vi "RSZVB Trace Response Data Error.vi"(8 "error in (no error)":errorcluster {"code" format="%.0x"}, 9 "Error Term (1)":i32=1, 10 "Channel (Trace) (1)":i32=1, 11 "VISA session":refnum<visa-resource-name>) -> (0 "error out":errorcluster {"code" format="%.0x"}, 1 "Trace Data":dbl[](array[numeric]) format="%^.3e", 3 "dup VISA session":refnum<visa-resource-name>)   [LabVIEW 2011]
doc: "This VI reads the current response values of the active data trace or memory trace.\n\nRemote-control command(s):\nFORMat[:DATA] REAL ,32\nCALCulate<Ch/Tr>:DATA? SCORr1 | ... | SCORr27"
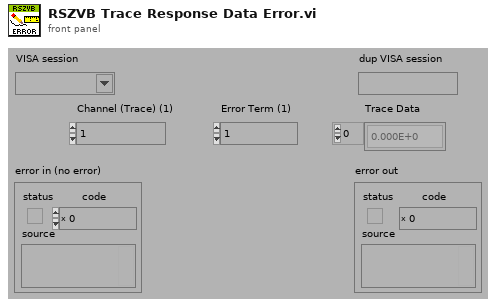
[diagram p1: front panel]
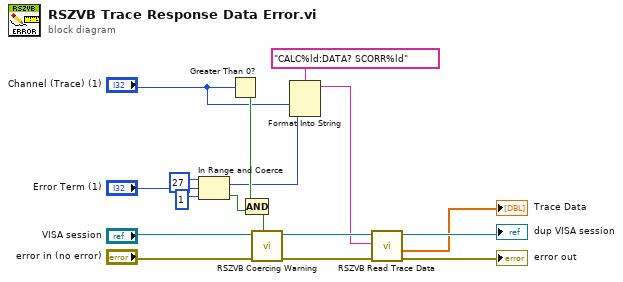
[diagram p0: block diagram]
diagram:
  n1 = In Range and Coerce(upper limit=27, x="Error Term (1)", lower limit=1) -> (coerced(x)=w1:i32, In Range?=w14:bool)
  n2 = Greater Than 0?(x="Channel (Trace) (1)") -> (x > 0?=w15:bool)
  n3 = Compound Arithmetic op=AND(w15, w14) -> (w16:bool)
  n4 = call "RSZVB Coercing Warning.vi"("In Range?"=w16, "error in (no error)"="error in (no error)", "VISA session"="VISA session") -> ("error out"=w13:errorcluster, "dup VISA session"=w12:refnum<visa-resource-name>)  [unwired: 7 in]
  n5 = Format Into String(format string="CALC%ld:DATA? SCORR%ld", "Channel (Trace) (1)", w1) -> (resulting string=w9:string)  [unwired: 2 in, 1 out]
  n6 = call "RSZVB Read Trace Data.vi"("error in (no error)"=w13, "Buffer"=w9, "VISA session"=w12) -> ("error out"=→"error out":errorcluster, "Trace Data"=→"Trace Data":dbl[], "dup VISA session"=→"dup VISA session":refnum<visa-resource-name>)  [unwired: 6 in]
